vi "Clear Selection.vi"(8 "Dates In":refnum<vi>) -> ()   [LabVIEW 2019, in "Custom Calendar.xctl"]
uses:
  Custom Calendar.xctl
  <vilib>/Utility/miscctls.llb/LVRowAndColumnTypeDef.ctl
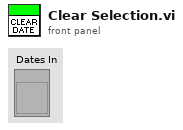
[diagram p1: front panel]
types:
  T1 = typedef "LVRowAndColumnTypeDef.ctl" = cluster{"Row":i32, "Column":i32}
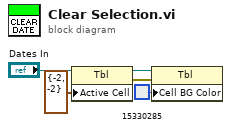
[diagram p0: block diagram]
diagram:
  n1 = property class="Tbl"(reference="Dates In", "Active Cell"=T1 {"Row"=-2, "Column"=-2} ("Active Cell:Active Cell")) -> (reference out=w3:refnum<vi>, error out=w2:errorcluster)  [unwired: 1 in]
  n2 = property class="Tbl"(reference=w3, error in=w2, "Cell BG Color"=u32 15330285 ("Active Cell:Cell Background Color")) -> ()  [unwired: 2 out]
